vi "SET_TemplateClass.vi"(8 "error in (no error)":errorcluster, 10 "Icon Framework.lvclass":refnum<class "Icon Framework.lvclass">, 11 "Icon.lvclass in":refnum<class "Icon.lvclass">) -> (0 "error out":errorcluster, 3 "Icon.lvclass out":refnum<class "Icon.lvclass">)   [LabVIEW 2020, in "Icon.lvclass"]
doc: "Specifies the Template Layer class."
uses:
  <vilib>/LabVIEW Icon API/lv_icon/Classes/Icon/Icon.lvclass
  <vilib>/LabVIEW Icon API/lv_icon/Classes/Icon Framework/Icon Framework.lvclass
  <vilib>/LabVIEW Icon API/lv_icon/Classes/Icon/Icon.lvclass/Icon.ctl
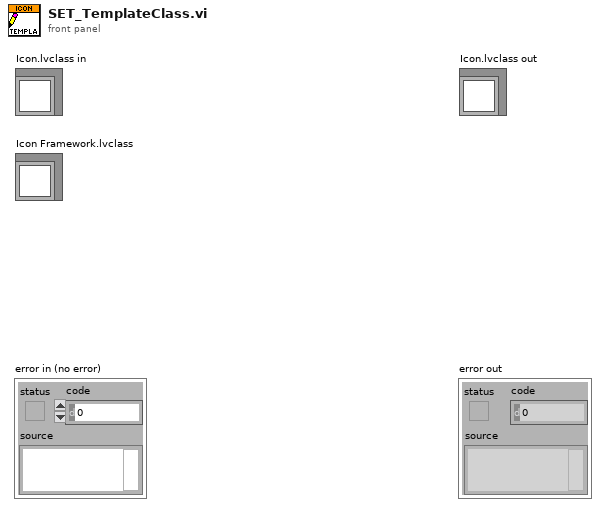
[diagram p1: front panel]
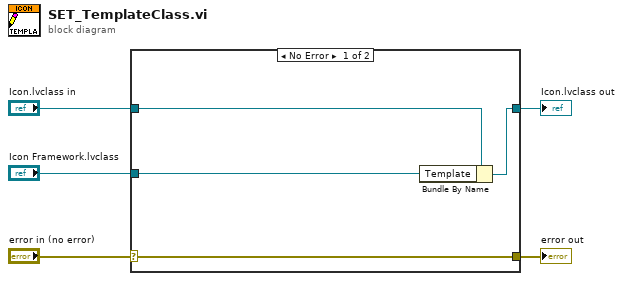
[diagram p0: block diagram]
diagram:
  n1 = case shown="No Error" "error in (no error)" {
    selector: "error in (no error)" -> [w9 w10]
    tunnel: [w9 w10] -> w4
    tunnel: [w7 w11] -> w2
    tunnel: "Icon.lvclass in" -> [w8 w11]
    tunnel: "Icon Framework.lvclass" -> [w6 _]
    frame No Error {
      n2 = Bundle By Name(cluster=w8, "Template"=w6) -> (w7:refnum<class "Icon.lvclass">)
    }
    frame Error {
    }
  }
  "error out" <- w4
  "Icon.lvclass out" <- w2
